vi "getData.vi"(8 "error in (no error)":errorcluster, 11 "PlayFile in":refnum<class "PlayFile.lvclass">) -> (0 "error out":errorcluster, 1 "dataType":T1(ring), 2 "data":T2, 3 "PlayFile out":refnum<class "PlayFile.lvclass">)   [LabVIEW 2011, in "Tools.lvlib" / "Scripting.lvlib" / "PlayFile.lvclass"]
uses:
  PlayFile.lvclass
  DatabaseHelpers/Database Objects/Channel/Channel.lvclass
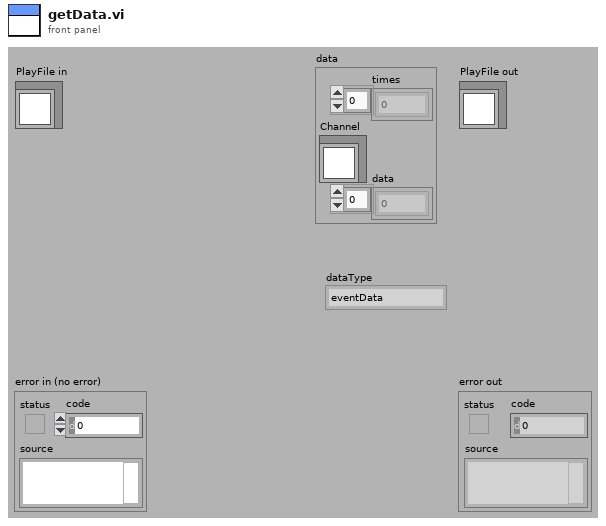
[diagram p1: front panel]
types:
  T1 = enum16{"eventData", "singleToneData", "fileData"}
  T2 = cluster{"times":dbl[], "Channel":refnum<class "Channel.lvclass">, "data":dbl[]}
  T3 = cluster{dbl[], "Channel.lvclass out":refnum<class "Channel.lvclass">, dbl[]}
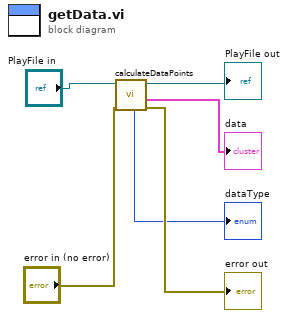
[diagram p0: block diagram]
diagram:
  n1 = call "calculateDataPoints.vi"("error in (no error)"="error in (no error)", "PlayFile in"="PlayFile in") -> ("error out"=→"error out":errorcluster, "Data"=→"data":T3, "PlayFile out"=→"PlayFile out":refnum<class "PlayFile.lvclass">, "dataType"=→"dataType":T1)  [unwired: 5 in, 1 out]
